vi "Add_Plugin_label.vi"(1 "Title in":string="1:2:3:4") -> (0 "Title out":string)   [LabVIEW 2011]
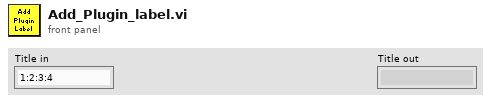
[diagram p1: front panel]
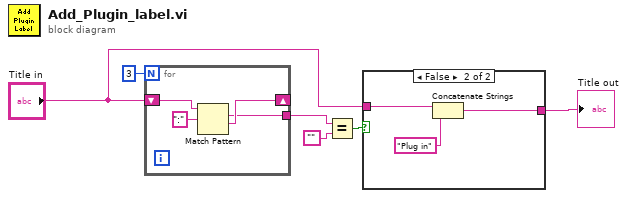
[diagram p0: block diagram]
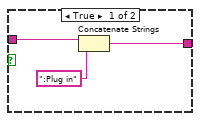
[diagram p2: hidden frame]
diagram:
  n1 = for {
    N: 3 -> [_]
    shift-right: [w8] -> _
    shift-left: "Title in" -> [w9]
    tunnel: [w7] -> w5
    n2 = Match Pattern(string=w9, regular expression=":") -> (match substring=w7:string, after substring=w8:string)  [unwired: 1 in, 2 out]
  }
  n3 = Equal?(x=w5, y="") -> (x = y?=w3:bool)
  n4 = case shown="False" w3 {
    tunnel: "Title in" -> [w13 w16]
    tunnel: [w11 w14] -> w2
    frame True {
      n5 = Concatenate Strings(w13, ":Plug in" ("Substring")) -> (w11:string)
    }
    frame False {
      n6 = Concatenate Strings(w16, "Plug in" ("Substring")) -> (w14:string)
    }
  }
  "Title out" <- w2
